vi "Tek_Read.vi"(8 "error in (no error)":errorcluster, 11 "VISA Refnum in":refnum<visa-resource-name>) -> (0 "error out":errorcluster, 1 "range":T1, 2 "Scope":cluster{dbl, dbl, dbl[]}(graph), 3 "VISA Refnum out":refnum<visa-resource-name>)   [LabVIEW 2022 SP3]
panel:
  out "data":dbl[](array[numeric])
  out "YOffset":dbl
  out "XZero":dbl
  out "YZero":dbl
  out "YMult":dbl
  out "XMult":dbl
  out "s/div":dbl
  out "V/div":dbl
  out "array":string[](array[string])
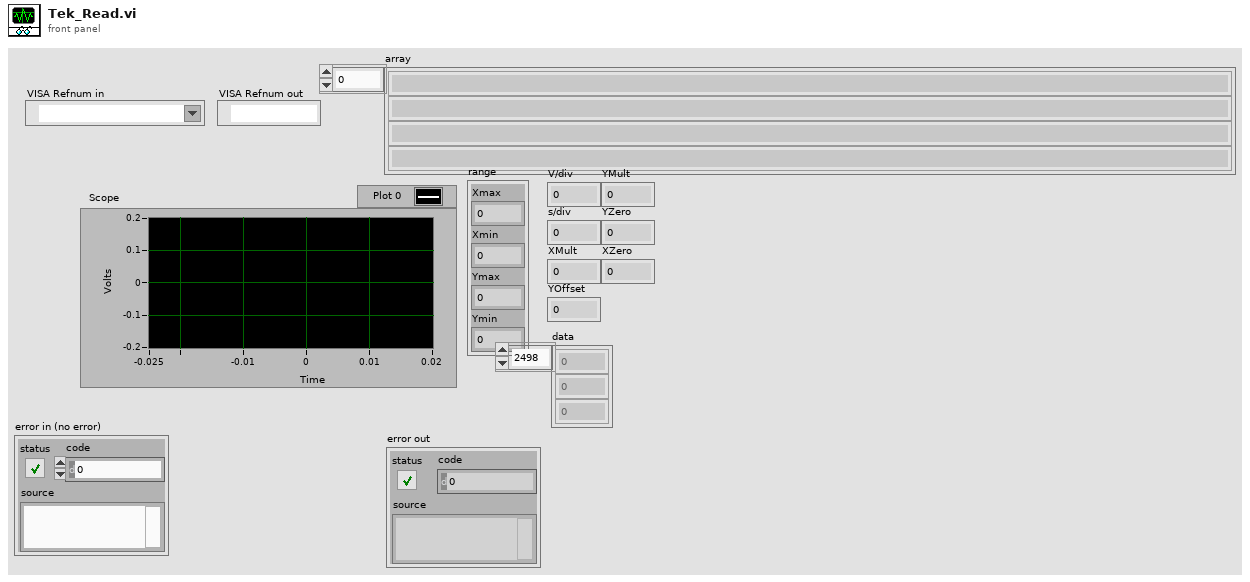
[diagram p1: front panel]
types:
  T1 = cluster{"Xmax":dbl, "Xmin":dbl, "Ymax":dbl, "Ymin":dbl}
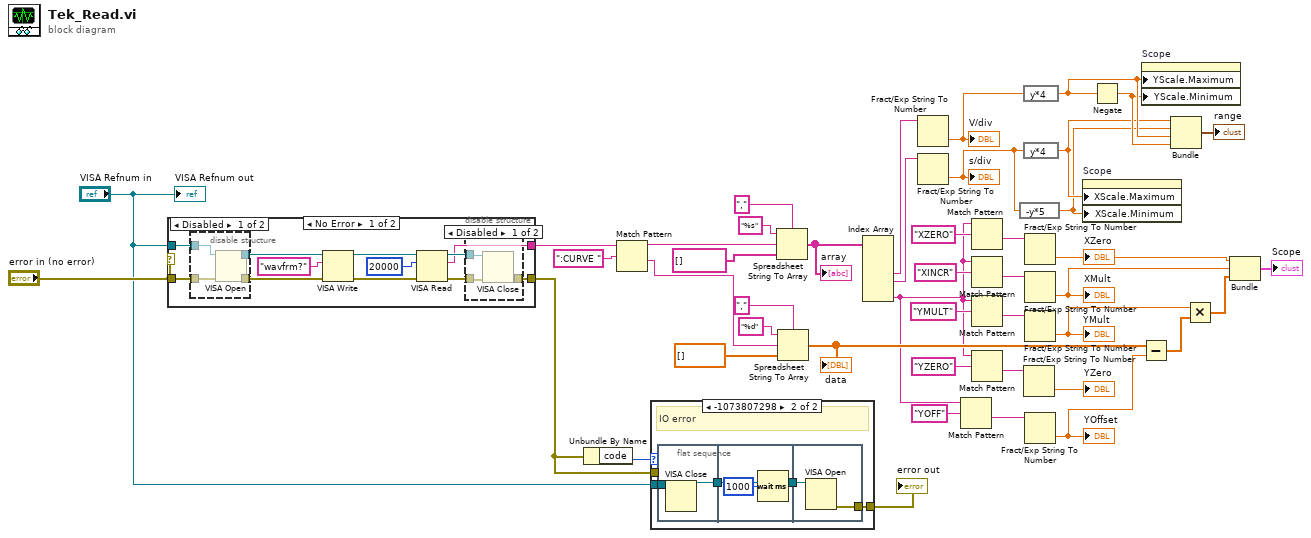
[diagram p0: block diagram]
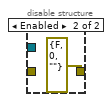
[diagram p3: hidden frame]
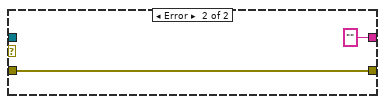
[diagram p5: hidden frame]
diagram:
  n1 = case shown="No Error" "error in (no error)" {
    tunnel: [w49 w69] -> w1
    tunnel: [w46 "" ("read buffer")] -> w44
    tunnel: "VISA Refnum in" -> [w52 _]
    tunnel: "error in (no error)" -> [w53 w69]
    frame No Error {
      n2 = disable-structure shown="Disabled" {
        disable-tunnel: w53 -> [w65 w66]
        disable-tunnel: w52 -> [w64 w67]
        disable-tunnel: [w63 w66] -> w51
        disable-tunnel: [w62 w67] -> w50
        frame Disabled {
          n3 = VISA Open(error in (no error)=w65, VISA resource name=w64) -> (VISA resource name=w62:refnum<visa-resource-name>, error out=w63:errorcluster)  [unwired: 3 in]
        }
        frame Enabled {
        }
      }
      n4 = VISA Write(VISA resource name=w50, write buffer="wavfrm?", error in (no error)=w51) -> (VISA resource name out=w56:refnum<visa-resource-name>, error out=w55:errorcluster)  [unwired: 1 out]
      n5 = VISA Read(VISA resource name=w56, byte count=u32 20000, error in (no error)=w55) -> (VISA resource name out=w47:refnum<visa-resource-name>, read buffer=w46:string, error out=w48:errorcluster)  [unwired: 1 out]
      n6 = disable-structure shown="Disabled" {
        disable-tunnel: [w60 errorcluster {"status"=FALSE, "code"=0, "source"=""} ("error out")] -> w49
        disable-tunnel: w48 -> [w59 _]
        disable-tunnel: w47 -> [w58 _]
        frame Disabled {
          n7 = VISA Close(VISA resource name=w58, error in (no error)=w59) -> (error out=w60:errorcluster)
        }
        frame Enabled {
        }
      }
    }
    frame Error {
    }
  }
  n8 = Unbundle By Name(w1) -> ("code"=w4:i32)
  n9 = Match Pattern(string=w44, regular expression=":CURVE ") -> (before substring=w12:string, after substring=w11:string)  [unwired: 1 in, 2 out]
  n10 = case shown="-1073807298" w4 {
    tunnel: "VISA Refnum in" -> [_ w74]
    tunnel: [w70 w71] -> w2
    tunnel: w1 -> [w70 _]
    frame Default {
    }
    frame -1073807298 {
      # "IO error"
      n11 = flat-sequence {
        tunnel: w74 -> [w75]
        tunnel: [w75] -> w73
        tunnel: w73 -> [w77]
        tunnel: [w77] -> w72
        tunnel: w72 -> [w79]
        tunnel: [w78] -> w71
        frame #0 {
          n12 = VISA Close(VISA resource name=w75) -> ()  [unwired: 1 in, 1 out]
        }
        frame #1 {
          n13 = Wait (ms)(milliseconds to wait=u32 1000) -> ()  [unwired: 1 out]
        }
        frame #2 {
          n14 = VISA Open(VISA resource name=w79) -> (error out=w78:errorcluster)  [unwired: 4 in, 1 out]
        }
      }
    }
  }
  "error out" <- w2
  n15 = Spreadsheet String To Array(delimiter (Tab)=",", format string="%s", spreadsheet string=w12, array type (2D Dbl)=string[] []) -> (array=w37:string[])
  "array" <- w37
  n16 = Spreadsheet String To Array(delimiter (Tab)=",", format string="%d", spreadsheet string=w11, array type (2D Dbl)=dbl[] []) -> (array=w26:dbl[])
  "data" <- w26
  n17 = Index Array(array=w37) -> (element #3=w36:string, element #4=w35:string, element #6=w17:string)  [unwired: 6 in, 3 out]
  n18 = Fract/Exp String To Number(string=w36) -> (number=w15:dbl)  [unwired: 3 in, 1 out]
  "V/div" <- w15
  n19 = Fract/Exp String To Number(string=w35) -> (number=w14:dbl)  [unwired: 3 in, 1 out]
  "s/div" <- w14
  n20 = Match Pattern(string=w17, regular expression="YOFF") -> (after substring=w19:string)  [unwired: 1 in, 3 out]
  n21 = Match Pattern(string=w17, regular expression="XZERO") -> (after substring=w28:string)  [unwired: 1 in, 3 out]
  n22 = Match Pattern(string=w17, regular expression="XINCR") -> (after substring=w33:string)  [unwired: 1 in, 3 out]
  n23 = Match Pattern(string=w17, regular expression="YMULT") -> (after substring=w32:string)  [unwired: 1 in, 3 out]
  n24 = Match Pattern(string=w17, regular expression="YZERO") -> (after substring=w29:string)  [unwired: 1 in, 3 out]
  n25 = expression code="-y*5"(w14) -> (w6:dbl)
  n26 = expression code="y*4"(w15) -> (w9:dbl)
  n27 = expression code="y*4"(w14) -> (w7:dbl)
  n28 = Fract/Exp String To Number(string=w29) -> (number=→"YZero":dbl)  [unwired: 3 in, 1 out]
  n29 = Fract/Exp String To Number(string=w28) -> (number=w22:dbl)  [unwired: 3 in, 1 out]
  "XZero" <- w22
  n30 = Fract/Exp String To Number(string=w33) -> (number=w21:dbl)  [unwired: 3 in, 1 out]
  "XMult" <- w21
  n31 = Fract/Exp String To Number(string=w32) -> (number=w23:dbl)  [unwired: 3 in, 1 out]
  "YMult" <- w23
  n32 = Fract/Exp String To Number(string=w19) -> (number=w16:dbl)  [unwired: 3 in, 1 out]
  "YOffset" <- w16
  n33 = property on="Scope" class="WFGraph (strict)"("XScale.Maximum"=w7, "XScale.Minimum"=w6) -> ()  [unwired: 2 in, 2 out]
  n34 = Negate(x=w9) -> (-x=w8:dbl)
  n35 = Subtract(x=w26, y=w16) -> (x-y=w24:dbl[])
  n36 = property on="Scope" class="WFGraph (strict)"("YScale.Maximum"=w9, "YScale.Minimum"=w8) -> ()  [unwired: 2 in, 2 out]
  n37 = Bundle(w7, w6, w9, w8) -> (→"range":cluster{dbl, dbl, dbl, dbl})  [unwired: 1 in]
  n38 = Multiply(x=w23, y=w24) -> (x*y=w20:dbl[])
  n39 = Bundle(w22, w21, w20) -> (→"Scope":cluster{dbl, dbl, dbl[]})  [unwired: 1 in]
  "VISA Refnum out" <- "VISA Refnum in"
